vi "LED Tester.vi"() -> ()   [LabVIEW 2017]
panel:
  in  "LED":enum8{"Red", "UV", "Green", "Blue"}(ring)
  in  "LED On/Off":bool
  in  "LED Power (mW)":dbl min=0.0 max=120.0 step=1.0
  in  "stop":bool
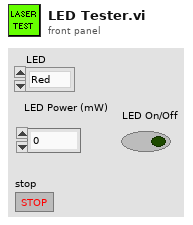
[diagram p1: front panel]
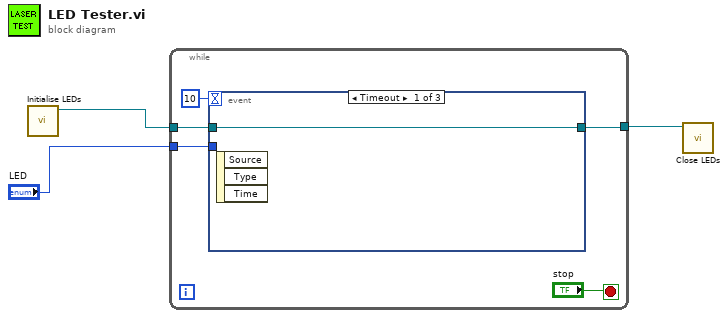
[diagram p0: block diagram]
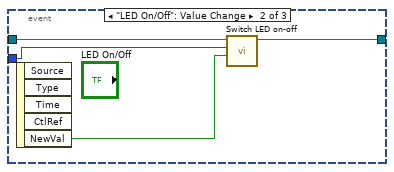
[diagram p2: hidden frame]
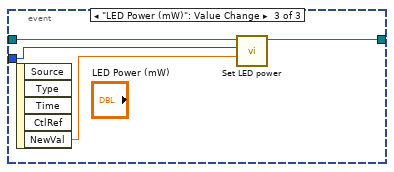
[diagram p3: hidden frame]
diagram:
  n1 = call "Initialise LEDs.vi"() -> ("LED handle"=w3:refnum<visa-resource-name>)  [unwired: 10 in, 1 out]
  n2 = while {
    tunnel: w3 -> [w7]
    tunnel: [w6] -> w1
    tunnel: "LED" -> [w4]
    stop <- "stop" stop-if-true
    n3 = event shown="[0] Timeout" {
      selector: _ -> [_ _ _]
      dyn-events: _ -> [_ _ _]
      timeout: 10 -> [_ _ _]
      tunnel: w7 -> [w9 w11 w17]
      tunnel: [w9 w10 w16] -> w6
      tunnel: w4 -> [_ w12 w14]
      event Timeout {
        n4 = event-data() -> ()  [unwired: 1 in, 3 out]
      }
      event "LED On/Off": Value Change {
        n5 = event-data() -> ("NewVal"=w13:bool)  [unwired: 1 in, 4 out]
        n6 = call "Switch LED on-off.vi"("LED On/Off"=w13, "LED"=w12, "LED handle in"=w11) -> ("LED handle out"=w10:refnum<visa-resource-name>)  [unwired: 7 in, 1 out]
      }
      event "LED Power (mW)": Value Change {
        n7 = event-data() -> ("NewVal"=w15:dbl)  [unwired: 1 in, 4 out]
        n8 = call "Set LED power.vi"("LED Power (%)"=w15, "LED"=w14, "LED handle in"=w17) -> ("LED handle out"=w16:refnum<visa-resource-name>)  [unwired: 7 in, 1 out]
      }
    }
  }
  n9 = call "Close LEDs.vi"("LED handle"=w1) -> ()  [unwired: 10 in, 1 out]
